vi "CreateDataGroups.vi"(8 "error in (no error)":errorcluster) -> (0 "error out":errorcluster)   [LabVIEW 2017]
uses:
  <vilib>/addons/PointValueMap/PointValueMap.lvlib
  <vilib>/addons/InsightCM/Utilities/GlobalConfiguration/GlobalConfiguration.lvlib
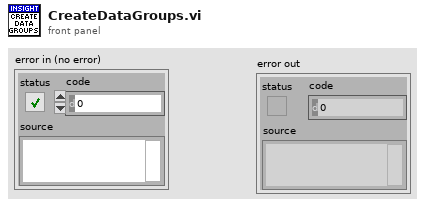
[diagram p1: front panel]
types:
  T1 = typedef "R2_Device.ctl" = cluster{"Id":string, "Name":string, "DeviceType":string, "HardwareName":string, "IpAddress":string, "HardwareInfo":T2[], "ApplicationType":string, "ApplicationVersion":string, "EquipmentIds":string[], "ConfigurationVersion":string, "State":T3, "Properties":T2[], "DataGroups":T4[], "BurstModeTrigger":T8}
  T2 = typedef "KeyValuePair.ctl" = cluster{"Key":string, "Value":string}
  T3 = typedef "DeviceState.ctl" = cluster{"Disabled":bool}
  T4 = typedef "R2_DataGroup.ctl" = cluster{"Name":string, "OperatingStates":T5[], "Properties":T2[], "EquipmentIds":string[], "AssetNodeId":string}
  T5 = typedef "OperatingState.ctl" = cluster{"Name":string, "Properties":T2[], "Triggers":T6[]}
  T6 = typedef "Trigger.ctl" = cluster{"Type":string, "Expression":string, "Conditions":T7[]}
  T7 = typedef "Condition.ctl" = cluster{"Source":string, "Type":string, "Operator":string, "CompareTo":string, "DwellSeconds":dbl}
  T8 = typedef "BurstModeTrigger.ctl" = cluster{"Trigger":T6, "SampleRate":string, "AcquisitionLength":string}
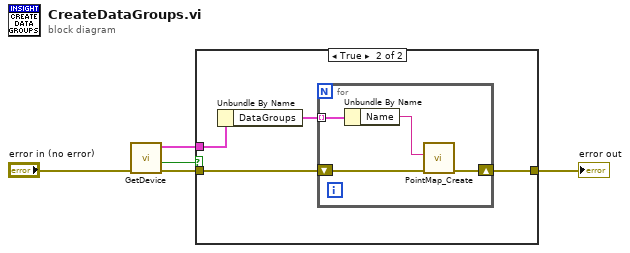
[diagram p0: block diagram]
diagram:
  n1 = call <vilib>:"GetDevice.vi"("error in (no error)"="error in (no error)") -> ("error out"=w2:errorcluster, "found"=w5:bool, "device configuration"=w3:T1)  [unwired: 8 in]
  n2 = case shown="True" w5 {
    tunnel: w3 -> [_ w10]
    tunnel: w2 -> [w6 w9]
    tunnel: [w6 w8] -> w1
    frame False {
    }
    frame True {
      n3 = Unbundle By Name(w10) -> ("DataGroups"=w7:T4[])
      n4 = for {
        shift-right: [w13] -> w8
        shift-left: w9 -> [w14]
        tunnel: w7 -> [w12] mode=indexing
        n5 = Unbundle By Name(w12) -> ("Name"=w11:string)
        n6 = call <vilib>:"PointMap_Create.vi"("error in (no error)"=w14, "Name"=w11) -> ("error out"=w13:errorcluster)  [unwired: 8 in, 1 out]
      }
    }
  }
  "error out" <- w1
